vi "Close_Connections.vi"(8 "Write Error in":errorcluster, 9 "Read Error in":errorcluster, 11 "AccelNET.lvlib:TCP.lvclass":refnum<class "TCP.lvclass">) -> (0 "Write Error Out":errorcluster, 1 "Read Error Out":errorcluster, 3 "AccelNET.lvlib:TCP.lvclass 2":refnum<class "TCP.lvclass">)   [LabVIEW 2012, in "AccelNET.lvlib" / "TCP.lvclass"]
uses:
  TCP.lvclass
  TCP.lvclass/TCP.ctl
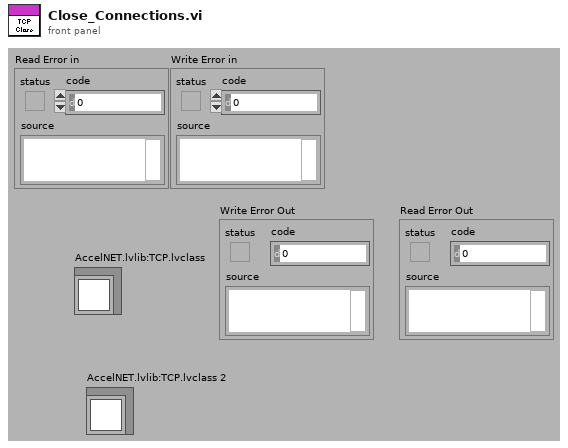
[diagram p1: front panel]
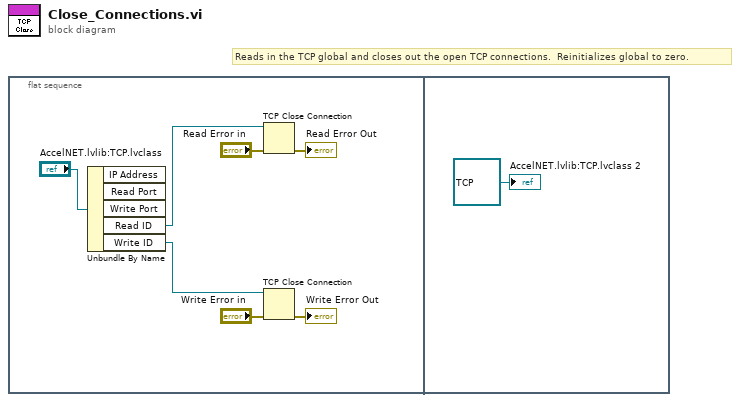
[diagram p0: block diagram]
diagram:
  # "Reads in the TCP global and closes out the open TCP connections.  Reinitializes global to zero."
  n1 = flat-sequence {
    frame #0 {
      n2 = Unbundle By Name("AccelNET.lvlib:TCP.lvclass") -> ("Read ID"=w2:refnum<k5>, "Write ID"=w1:refnum<k5>)  [unwired: 3 out]
      n3 = TCP Close Connection(connection ID=w2, error in (no error)="Read Error in") -> (error out=→"Read Error Out":errorcluster)  [unwired: 1 in, 1 out]
      n4 = TCP Close Connection(connection ID=w1, error in (no error)="Write Error in") -> (error out=→"Write Error Out":errorcluster)  [unwired: 1 in, 1 out]
    }
    frame #1 {
      "AccelNET.lvlib:TCP.lvclass 2" <- refnum<class "TCP.lvclass"> refnum ("AccelNET.lvlib:TCP.lvclass 2")
    }
  }
